vi "CircleAnalysis.vi"(11 "Cluster":T1 {"r" format="%.6f"}) -> ()   [LabVIEW 2022 SP3]
panel:
  out "Intensity Graph":dbl[][](graph)
  out "best fit":cluster{"theta_r":dbl, "w_r":dbl}
  out "circle center":cluster{"x_0":dbl, "y_0":dbl}
  out "Niquist":cluster{dbl[], dbl[]}[](graph)
  out "Waveform Graph":dbl[][](graph)
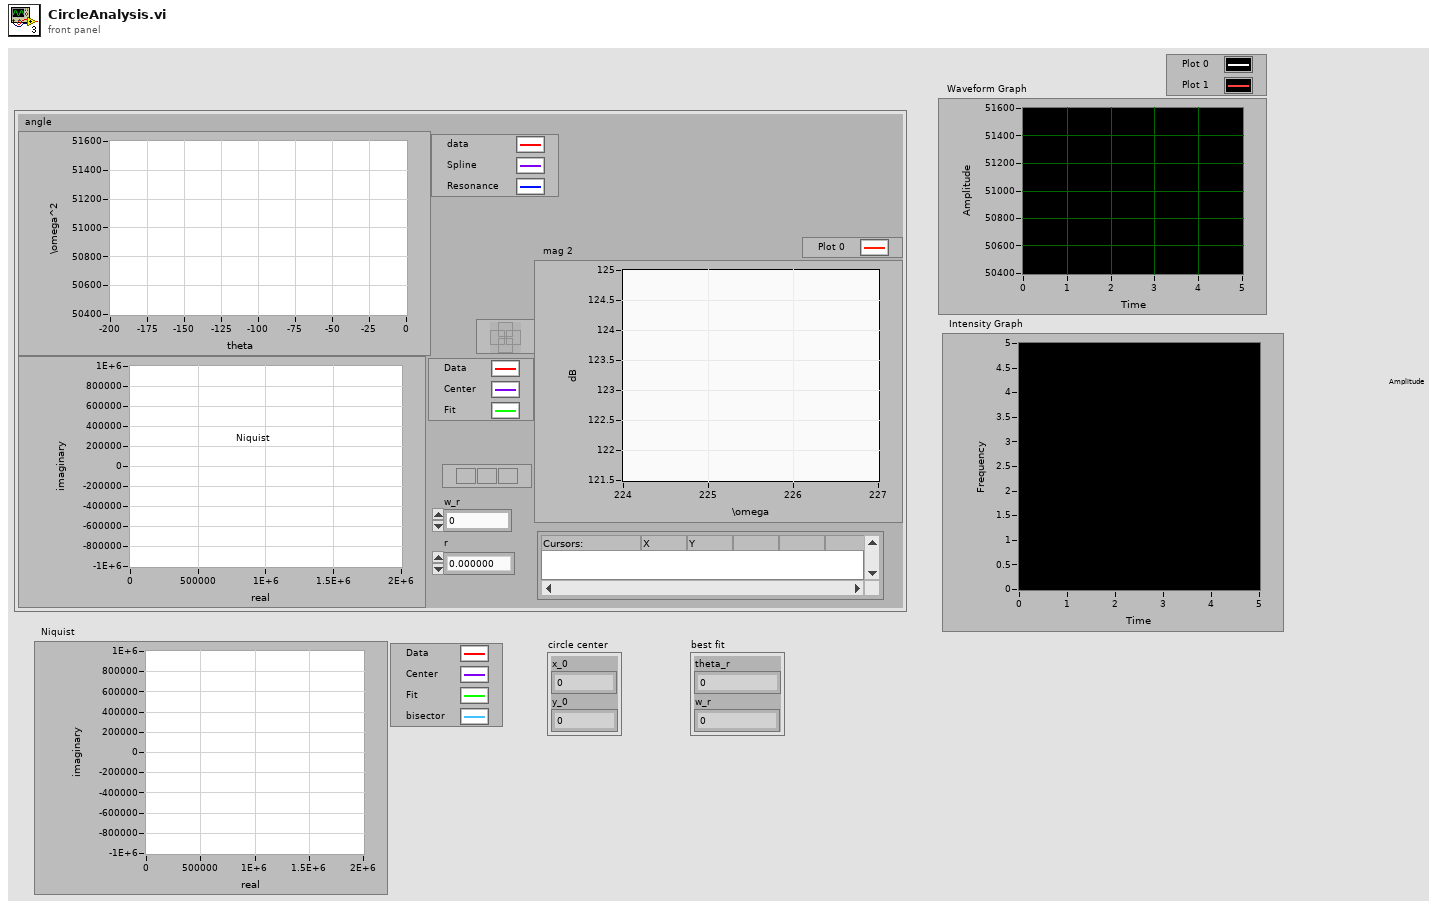
[diagram p1: front panel]
types:
  T1 = cluster{"angle":cluster{dbl[], "yi":dbl[]}[], "Niquist":cluster{dbl[], dbl[]}[], "mag 2":cluster{dbl[], dbl[]}, "w_r":dbl, "r":dbl}
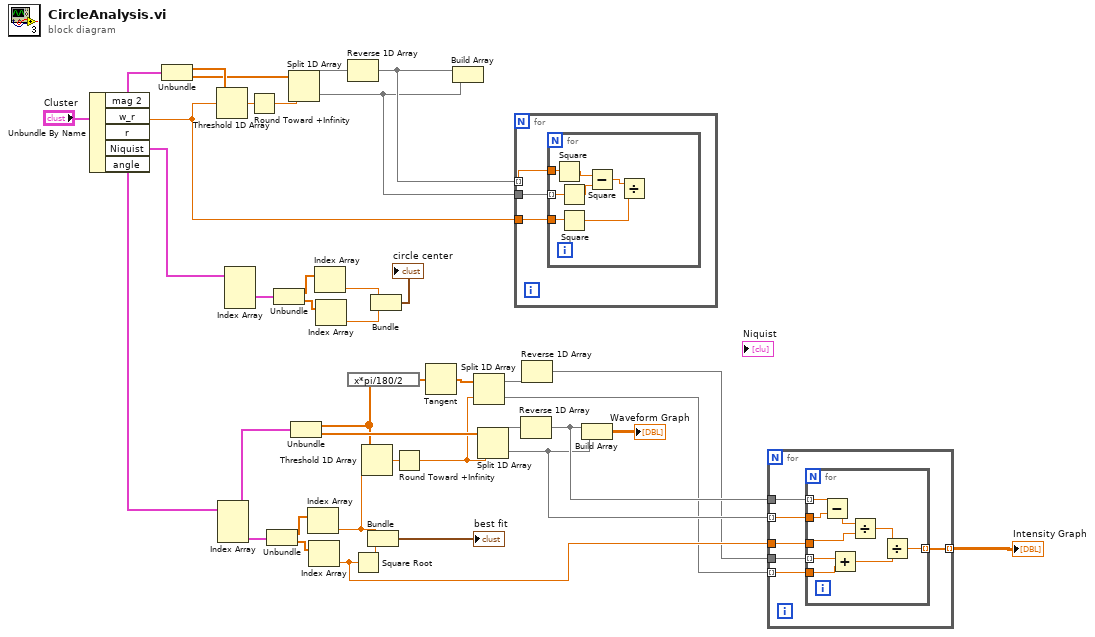
[diagram p0: block diagram]
diagram:
  n1 = Unbundle By Name("Cluster") -> ("mag 2"=w39:cluster{dbl[], dbl[]}, "w_r"=w31:dbl, "Niquist"=w30:cluster{dbl[], dbl[]}[], "angle"=w24:cluster{dbl[], "yi":dbl[]}[])  [unwired: 1 out]
  n2 = Unbundle(w39) -> (w35:dbl[], w34:dbl[])
  n3 = Threshold 1D Array(2:w31, 3:w35) -> (0:w38:dbl)  [unwired: 1 in]
  n4 = Index Array(array=w24) -> (element #1=w14:cluster{dbl[], "yi":dbl[]}, element #3=w23:cluster{dbl[], "yi":dbl[]})  [unwired: 3 in, 1 out]
  n5 = Index Array(array=w30) -> (element #2=w29:cluster{dbl[], dbl[]})  [unwired: 3 in, 2 out]
  n6 = Round Toward +Infinity(x=w38) -> (ceil(x): smallest int >= x=w37:dbl)
  n7 = Unbundle(w23) -> (w25:dbl[], "yi"=w26:dbl[])
  n8 = Unbundle(w29) -> (w28:dbl[], w27:dbl[])
  n9 = Split 1D Array(array=w34, index=w37) -> (first subarray=w36:dbl[], second subarray=w32:dbl[])
  n10 = Unbundle(w14) -> (w5:dbl[], "yi"=w17:dbl[])
  n11 = Index Array(array=w25) -> (element=w13:dbl)  [unwired: 1 in]
  n12 = Index Array(array=w26) -> (element=w10:dbl)  [unwired: 1 in]
  n13 = Index Array(array=w28) -> (element=w21:dbl)  [unwired: 1 in]
  n14 = Index Array(array=w27) -> (element=w22:dbl)  [unwired: 1 in]
  n15 = Reverse 1D Array(array=w36) -> (reversed array=w33:dbl[])
  n16 = expression code="x*pi/180/2"(w5) -> (w4:dbl[])
  n17 = Square Root(x=w10) -> (sqrt(x)=w18:dbl)
  n18 = Threshold 1D Array(2:w13, 3:w5) -> (0:w15:dbl)  [unwired: 1 in]
  n19 = Bundle("Numeric"=w13, w18) -> (→"best fit":cluster{"Numeric":dbl, dbl})  [unwired: 1 in]
  n20 = Bundle(w21, w22) -> (→"circle center":cluster{dbl, dbl})  [unwired: 1 in]
  n21 = Round Toward +Infinity(x=w15) -> (ceil(x): smallest int >= x=w9:dbl)
  n22 = Tangent(1:w4) -> (0:w2:dbl[])
  n23 = Build Array(w33, w32) -> ()  [unwired: 1 out]
  n24 = Split 1D Array(array=w2, index=w9) -> (first subarray=w8:dbl[], second subarray=w6:dbl[])
  n25 = Split 1D Array(array=w17, index=w9) -> (first subarray=w16:dbl[], second subarray=w7:dbl[])
  n26 = for {
    tunnel: w33 -> [w42] mode=indexing
    tunnel: w32 -> [w43]
    tunnel: w31 -> [w41]
    n27 = for {
      tunnel: w43 -> [w49] mode=indexing
      tunnel: w42 -> [w50]
      tunnel: w41 -> [w45]
      n28 = Square(x=w50) -> (x^2=w48:dbl)
      n29 = Square(x=w49) -> (x^2=w46:dbl)
      n30 = Square(x=w45) -> (x^2=w44:dbl)
      n31 = Subtract(x=w48, y=w46) -> (x-y=w47:dbl)
      n32 = Divide(x=w47, y=w44) -> ()  [unwired: 1 out]
    }
  }
  n33 = Reverse 1D Array(array=w16) -> (reversed array=w11:dbl[])
  n34 = Reverse 1D Array(array=w8) -> (reversed array=w3:dbl[])
  n35 = Build Array(w11, w7) -> (→"Waveform Graph":dbl[][])
  n36 = for {
    tunnel: w11 -> [w56]
    tunnel: w7 -> [w55] mode=indexing
    tunnel: w10 -> [w54]
    tunnel: w6 -> [w53] mode=indexing
    tunnel: w3 -> [w52]
    tunnel: [w51] -> w1 mode=indexing
    n37 = for {
      tunnel: w56 -> [w64] mode=indexing
      tunnel: w55 -> [w65]
      tunnel: w54 -> [w62]
      tunnel: w53 -> [w60]
      tunnel: w52 -> [w61] mode=indexing
      tunnel: [w57] -> w51 mode=indexing
      n38 = Subtract(x=w64, y=w65) -> (x-y=w63:dbl)
      n39 = Add(x=w61, y=w60) -> (x+y=w58:dbl)
      n40 = Divide(x=w63, y=w62) -> (x/y=w59:dbl)
      n41 = Divide(x=w59, y=w58) -> (x/y=w57:dbl)
    }
  }
  "Intensity Graph" <- w1
